vi "UTF-8至文本转换.vi"(9 "文本 2":string, 11 "utf-8文本":string) -> (1 "utf-8文本 2":string, 3 "文本":string)   [LabVIEW 2015]
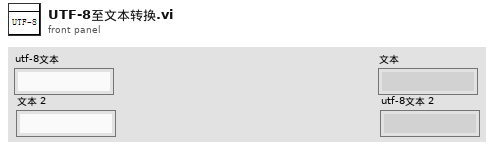
[diagram p1: front panel]
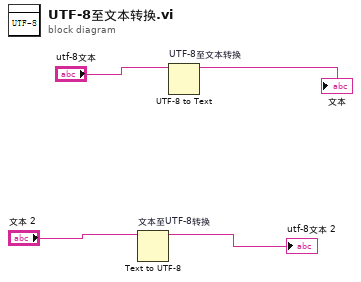
[diagram p0: block diagram]
diagram:
  n1 = Text to UTF-8 "文本至UTF-8转换"(11:"文本 2") -> (3:→"utf-8文本 2":string)  [unwired: 2 in, 1 out]
  n2 = UTF-8 to Text "UTF-8至文本转换"(11:"utf-8文本") -> (3:→"文本":string)  [unwired: 2 in, 1 out]
